vi "APP_FileReader.vi"(10 "file path (use dialog)":path) -> (2 "output byte stream":u8[](array[numeric]), 3 "path":path)   [LabVIEW 2014]
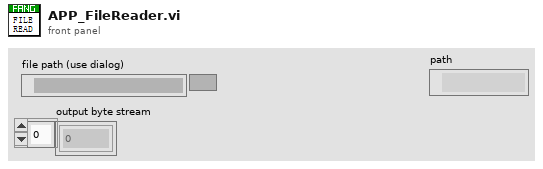
[diagram p1: front panel]
types:
  T1 = enum16{"open", "replace", "create", "open or create", "replace or create", "replace or create with confirmation"}
  T2 = enum16{"big-endian, network order", "native, host order", "little-endian"}
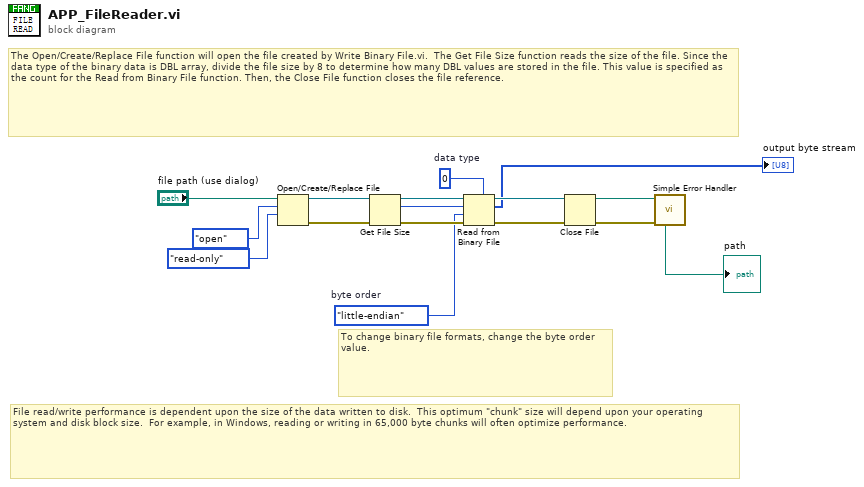
[diagram p0: block diagram]
diagram:
  w9 = T2."little-endian"  # byte order
  w10 = u8 0  # data type
  # "File read/write performance is dependent upon the size of the data written to disk.  This optimum \"chunk\" size will depend upon your operating system and disk block size.  For example, in Windows, reading or writing in 65,000 byte chunks will often optimize performance."
  # "To change binary file formats, change the byte order value."
  # "The Open/Create/Replace File function will open the file created by Write Binary File.vi.  The Get File Size function reads the size of the file. Since the data type of the binary data is DBL array, divide the file size by 8 to determine how many DBL values are stored in the file. This value is specified as the count for the Read from Binary File function. Then, the Close File function closes the file reference."
  n1 = Open/Create/Replace File(file path (use dialog)="file path (use dialog)", operation (0:open)=T1."open", access (0:read/write)=enum16{"read/write", "read-only", "write-only"}."read-only") -> (refnum out=w6:refnum<file>, error out=w7:errorcluster)  [unwired: 3 in, 1 out]
  n2 = Get File Size(file=w6, error in=w7) -> (refnum out=w15:refnum<file>, size (in bytes)=w3:i64, 0:w12:errorcluster)
  n3 = Read from Binary File(5:w10, 8:w12, 9:w9, 10:w3, 11:w15) -> (0:w13:errorcluster, 2:→"output byte stream":u8[], 3:w14:refnum<file>)  [unwired: 1 in, 1 out]
  n4 = Close File(refnum=w14, error in=w13) -> (path=→"path":path, error out=w5:errorcluster)
  n5 = call <vilib>:"Simple Error Handler.vi"("error in (no error)"=w5) -> ()  [unwired: 4 in, 5 out]
